vi "Test Read Numerics.vi"(11 "TwinCAT ADS in":refnum<class "TwinCAT ADS.lvclass">) -> (3 "TwinCAT ADS out":refnum<class "TwinCAT ADS.lvclass">)   [LabVIEW 2018]
uses:
  TwinCAT ADS Class/TwinCAT ADS.lvclass
  1ec89d4e-eb1f-4200-8905-b90c080105c4.vi
  585f919c-50ae-4d57-bc21-e4fdde987265.vi
  b37b65c8-3294-4411-875b-58a00d0f2e6b.vi
  4189af63-aa5f-45eb-a465-53f4a070e9db.vi
  75a96fe2-82aa-4a60-9f90-7314e7c3bfda.vi
  224d71c1-e242-4dba-8587-3d6bb118da48.vi
  8c23fba3-ff2e-429a-85b3-a2a5746d3602.vi
  d8ba1b3a-7848-44fd-b2b9-f7a4c8308b72.vi
  3c26fa66-3b82-4eae-ba6f-f4b83f5444f7.vi
  e7a7b24b-aede-49d7-b369-bb451e1de87e.vi
  TwinCAT ADS Class/VIs/Data/Read.vi
  <vilib>/addons/_JKI Toolkits/Caraya/classes/Assert/Assert Equal Value and Type_Variant.vi
  <vilib>/addons/_JKI Toolkits/Caraya/classes/Assert/Assert Equal Value_Variant.vi
  <vilib>/addons/_JKI Toolkits/Caraya/classes/Assert/Assert Almost Equal_Float.vi
  <vilib>/addons/_JKI Toolkits/Caraya/classes/Assert/Assert.lvclass
  <vilib>/addons/_JKI Toolkits/Caraya/classes/Test/Test.lvclass
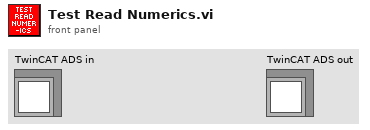
[diagram p1: front panel]
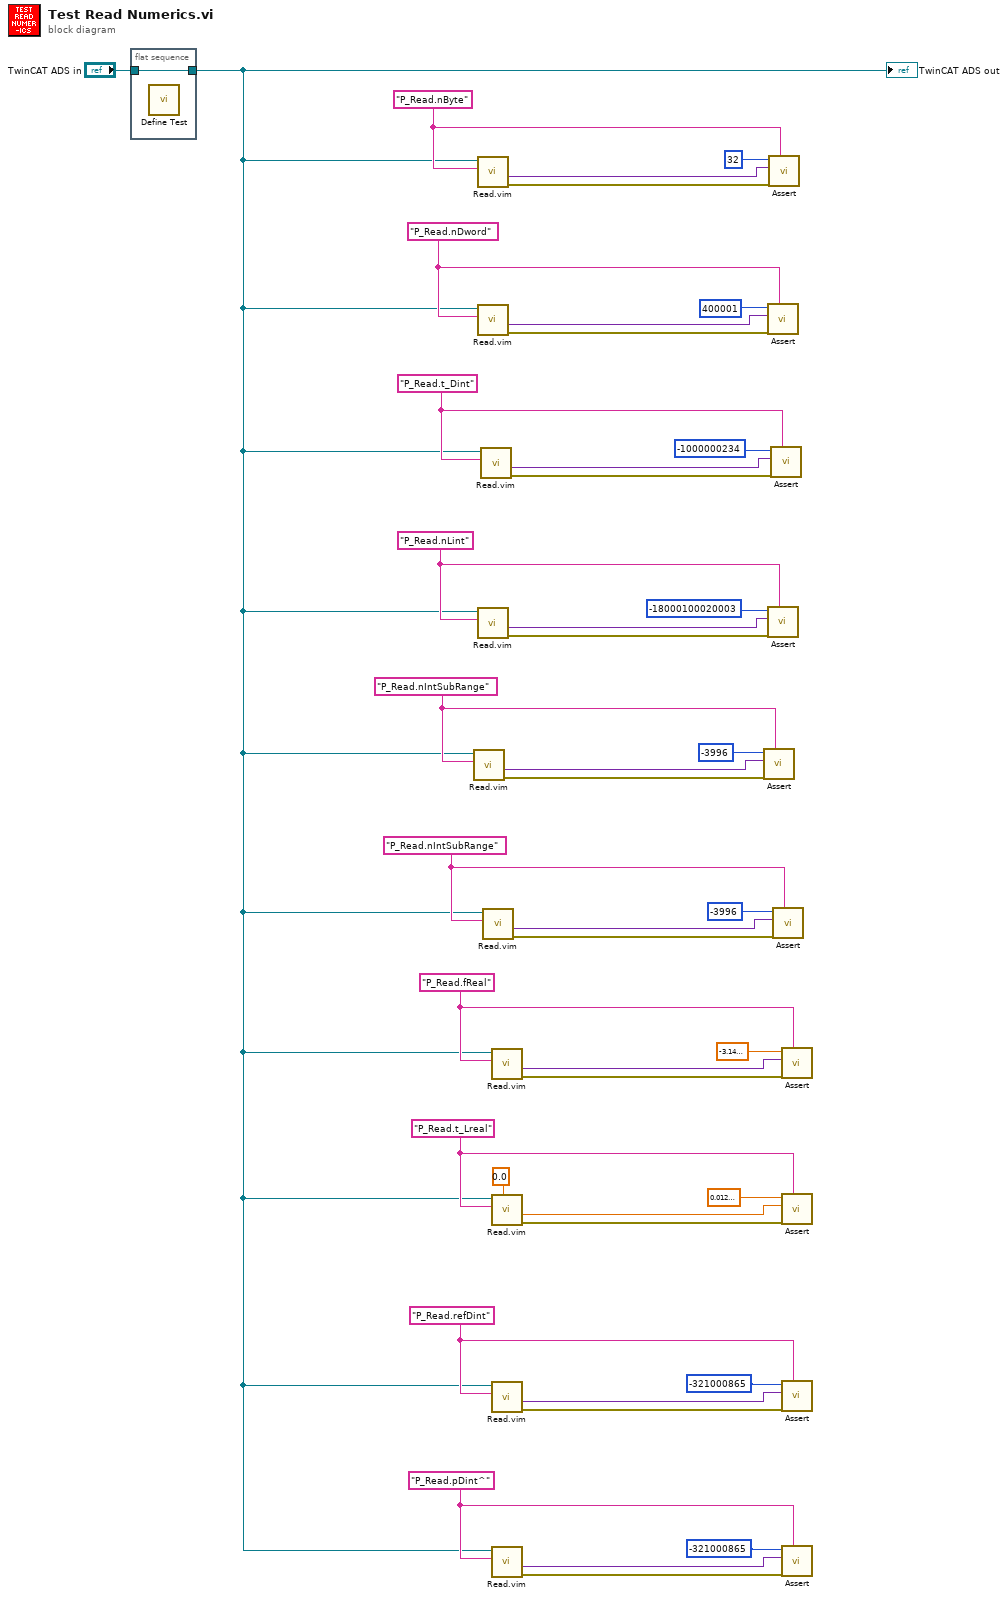
[diagram p0: block diagram]
diagram:
  w2 = "P_Read.pDint^" ("Symbol Name")
  w11 = "P_Read.refDint" ("Symbol Name")
  w12 = "P_Read.t_Lreal" ("Symbol Name")
  w20 = "P_Read.fReal" ("Symbol Name")
  w21 = "P_Read.t_Dint" ("Symbol Name")
  w27 = "P_Read.nIntSubRange" ("Symbol Name")
  w30 = "P_Read.nIntSubRange" ("Symbol Name")
  w31 = "P_Read.nLint" ("Symbol Name")
  w32 = "P_Read.nDword" ("Symbol Name")
  w33 = "P_Read.nByte" ("Symbol Name")
  n1 = flat-sequence {
    tunnel: "TwinCAT ADS in" -> [w44]
    tunnel: [w44] -> w1
    frame #0 {
      n2 = call <vilib>:"Define Test.vi"() -> ()  [unwired: 10 in, 2 out]
    }
  }
  n3 = call "Read.vim"("Symbol Name"=w30, "TwinCAT ADS in"=w1) -> ("error out"=w37:errorcluster, "Value"=w36:variant)  [unwired: 7 in, 1 out]
  n4 = call "Read.vim"("Symbol Name"=w33, "TwinCAT ADS in"=w1) -> ("error out"=w43:errorcluster, "Value"=w29:variant)  [unwired: 7 in, 1 out]
  n5 = call "Read.vim"("Symbol Name"=w32, "TwinCAT ADS in"=w1) -> ("error out"=w42:errorcluster, "Value"=w41:variant)  [unwired: 7 in, 1 out]
  n6 = call "Read.vim"("Symbol Name"=w31, "TwinCAT ADS in"=w1) -> ("error out"=w38:errorcluster, "Value"=w7:variant)  [unwired: 7 in, 1 out]
  n7 = call "Read.vim"("Symbol Name"=w21, "TwinCAT ADS in"=w1) -> ("error out"=w23:errorcluster, "Value"=w6:variant)  [unwired: 7 in, 1 out]
  n8 = call "Read.vim"("Symbol Name"=w27, "TwinCAT ADS in"=w1) -> ("error out"=w24:errorcluster, "Value"=w25:variant)  [unwired: 7 in, 1 out]
  n9 = call "Read.vim"("Symbol Name"=w20, "TwinCAT ADS in"=w1) -> ("error out"=w17:errorcluster, "Value"=w18:variant)  [unwired: 7 in, 1 out]
  n10 = call "Read.vim"("Type"=0.0, "Symbol Name"=w12, "TwinCAT ADS in"=w1) -> ("error out"=w16:errorcluster, "Value"=w14:dbl)  [unwired: 6 in, 1 out]
  n11 = call "Read.vim"("Symbol Name"=w11, "TwinCAT ADS in"=w1) -> ("error out"=w8:errorcluster, "Value"=w9:variant)  [unwired: 7 in, 1 out]
  n12 = call "Read.vim"("Symbol Name"=w2, "TwinCAT ADS in"=w1) -> ("error out"=w5:errorcluster, "Value"=w4:variant)  [unwired: 7 in, 1 out]
  n13 = call-poly <vilib>:"Assert.vi"("Label"=w30, "error in (no error)"=w37, "Y"=w36, "X"=i16 -3996) -> ()  [unwired: 6 in, 2 out]
  n14 = call-poly <vilib>:"Assert.vi"("Label"=w32, "error in (no error)"=w42, "Y"=w41, "X"=u32 400001) -> ()  [unwired: 6 in, 2 out]
  n15 = call-poly <vilib>:"Assert.vi"("Label"=w31, "error in (no error)"=w38, "Y"=w7, "X"=i64 -18000100020003) -> ()  [unwired: 6 in, 2 out]
  n16 = call-poly <vilib>:"Assert.vi"("Label"=w33, "error in (no error)"=w43, "Y"=w29, "X"=u8 32 ("Value")) -> ()  [unwired: 6 in, 2 out]
  n17 = call-poly <vilib>:"Assert.vi"("Label"=w21, "error in (no error)"=w23, "Y"=w6, "X"=-1000000234) -> ()  [unwired: 6 in, 2 out]
  n18 = call-poly <vilib>:"Assert.vi"("Label"=w27, "error in (no error)"=w24, "Y"=w25, "X"=i16 -3996) -> ()  [unwired: 6 in, 2 out]
  n19 = call-poly <vilib>:"Assert.vi"("Label"=w20, "error in (no error)"=w17, "Y"=w18, "X"=sgl -3.14) -> ()  [unwired: 6 in, 2 out]
  n20 = call-poly <vilib>:"Assert.vi"("Label"=w12, "error in (no error)"=w16, "Y"=w14, "X"=0.012000000104308128) -> ()  [unwired: 6 in, 2 out]
  n21 = call-poly <vilib>:"Assert.vi"("Label"=w11, "error in (no error)"=w8, "Y"=w9, "X"=-321000865) -> ()  [unwired: 6 in, 2 out]
  n22 = call-poly <vilib>:"Assert.vi"("Label"=w2, "error in (no error)"=w5, "Y"=w4, "X"=-321000865) -> ()  [unwired: 6 in, 2 out]
  "TwinCAT ADS out" <- w1
